vi "reaction_game.vi"() -> ()   [LabVIEW 2017]
panel:
  out "results (ms)":u32
  in  "?":bool
  out "message":string
  in  "pushbutton":bool
  out "indicator":bool
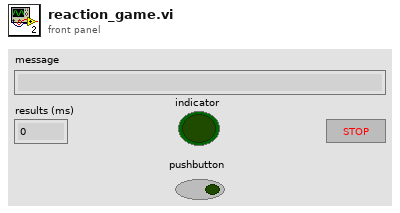
[diagram p1: front panel]
types:
  T1 = enum16{"Begin", "RandomWait", "WaitForReaction", "CalculateResults"}
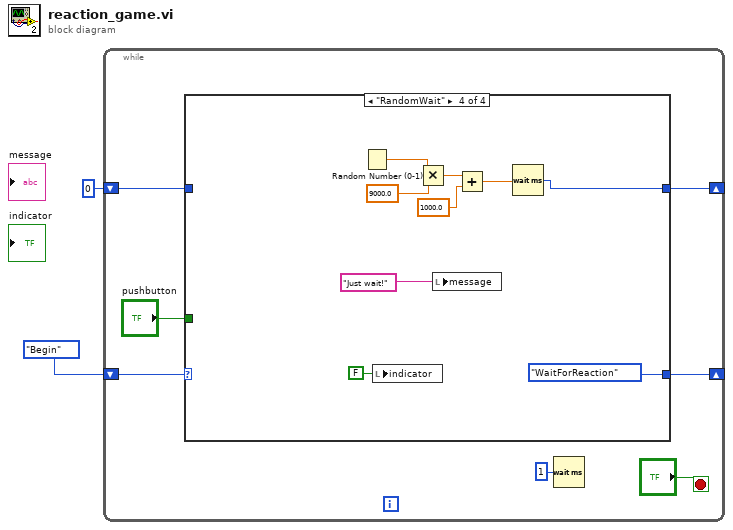
[diagram p0: block diagram]
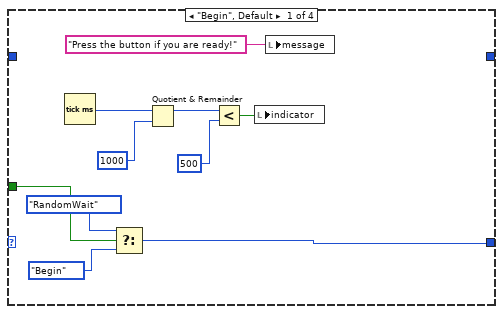
[diagram p2: hidden frame]
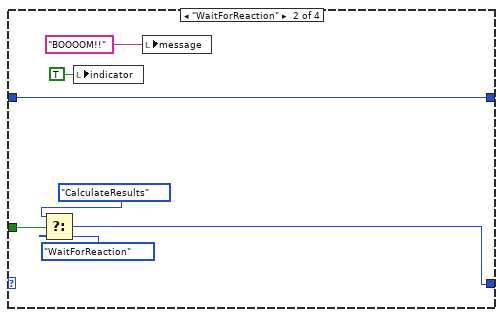
[diagram p3: hidden frame]
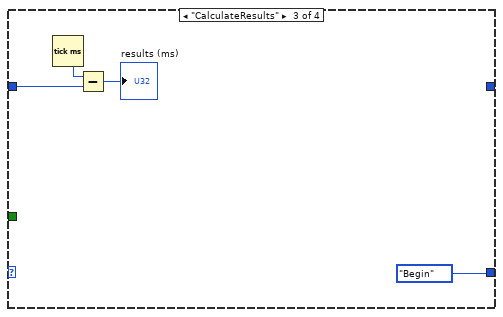
[diagram p4: hidden frame]
diagram:
  n1 = while {
    shift-right: [w6] -> _
    shift-left: T1."Begin" -> [w7]
    shift-right: [w4] -> _
    shift-left: u32 0 ("millisecond timer value") -> [w3]
    stop <- "?" stop-if-true
    n2 = case shown="\"RandomWait\"" w7 {
      tunnel: "pushbutton" -> [w13 w23 _ _]
      tunnel: [w10 w20 T1."Begin" T1."WaitForReaction"] -> w6
      tunnel: [_ w24 _ w32] -> w4
      tunnel: w3 -> [_ w24 w29 _]
      frame "Begin", Default {
        n3 = Tick Count (ms)() -> (millisecond timer value=w19:u32)
        n4 = Select(t=T1."RandomWait", s=w13, f=T1."Begin") -> (s? t:f=w10:T1)
        n5 = Quotient & Remainder(x=w19, y=i64 1000) -> (x-y*floor(x/y)=w18:i64)  [unwired: 1 out]
        n6 = Less?(x=w18, y=i64 500) -> (x < y?=w15:bool)
        n7 = local write "indicator"(w15) -> ()
        n8 = local write "message"("Press the button if you are ready!") -> ()
      }
      frame "WaitForReaction" {
        n9 = Select(t=T1."CalculateResults", s=w23, f=T1."WaitForReaction") -> (s? t:f=w20:T1)
        n10 = local write "indicator"(TRUE ("indicator")) -> ()
        n11 = local write "message"("BOOOOM!!" ("message")) -> ()
      }
      frame "CalculateResults" {
        n12 = Tick Count (ms)() -> (millisecond timer value=w30:u32)
        n13 = Subtract(x=w30, y=w29) -> (x-y=→"results (ms)":u32)
      }
      frame "RandomWait" {
        n14 = Random Number (0-1)() -> (number: 0 to 1=w39:dbl)
        n15 = local write "indicator"(FALSE ("indicator")) -> ()
        n16 = Multiply(x=w39, y=9000.0) -> (x*y=w36:dbl)
        n17 = local write "message"("Just wait!" ("message")) -> ()
        n18 = Add(x=w36, y=1000.0) -> (x+y=w33:dbl)
        n19 = Wait (ms)(milliseconds to wait=w33) -> (millisecond timer value=w32:u32)
      }
    }
    n20 = Wait (ms)(milliseconds to wait=u32 1) -> ()  [unwired: 1 out]
  }
